vi "Bug man temp globals.vi"() -> ()   [LabVIEW 2019]
doc: "Thise are the global variables for the bug experiment.\n\nThe \"exec\" cluster is under executive control, all other variables are under control of the DAQ state machine.\n\nPaul K Dxion\nP3600\nCSUSB Physics"
uses:
  typedefs/temp cont cluster.ctl
  typedefs/temp exec cluster.ctl
  typedefs/temp mode enum.ctl
  typedefs/temp indicator.ctl
  typedefs/temp cont utility.ctl
panel:
  in  "T cont":T1={"exec"={"T mode"=enum."Listening to exec", "man power"=0.5, "log"=FALSE}, "T status"={"Temp"=0.0, "Power"=0.0}, "utility"={"meas index"=0, "wait (ms)"=300, "H Vmax"=8.5, "power out"=0.0, "heat volt out"=0.0, "heat volt in"=0.0, "therm volt"=0.0, "t T P hist"=[]}} {"utility"."therm volt" format="%_6g"; "utility"."heat volt in" format="%_6g"; "utility"."heat volt out" format="%_6g"; "utility"."power out" format="%_6g"; "utility"."H Vmax" format="%_6g"; "exec"."man power" format="%_6g"; "T status"."Power" format="%_6g"; "T status"."Temp" format="%_6g"}
  # "exec, wait, and T params are under exec control"
  # "T status and the voltages are under DAQ state machine control"
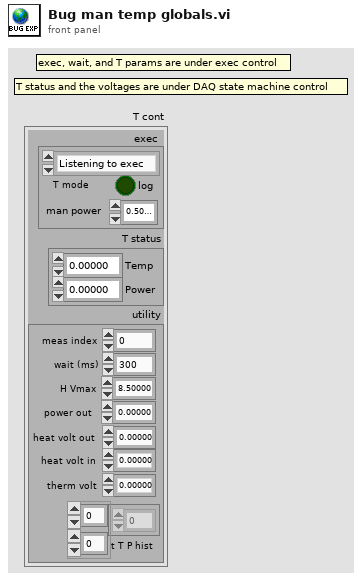
[diagram p1: front panel]
types:
  T1 = typedef "temp cont cluster.ctl" = cluster{"exec":T2, "T status":T4, "utility":T5}
  T2 = typedef "temp exec cluster.ctl" = cluster{"T mode":T3, "man power":dbl, "log":bool}
  T3 = typedef "temp mode enum.ctl" = enum16{"Setting up", "Listening to exec", "Exit"}
  T4 = typedef "temp indicator.ctl" = cluster{"Temp":dbl, "Power":dbl}
  T5 = typedef "temp cont utility.ctl" = cluster{"meas index":i32, "wait (ms)":i32, "H Vmax":dbl, "power out":dbl, "heat volt out":dbl, "heat volt in":dbl, "therm volt":dbl, "t T P hist":dbl[][]}
diagram:
